vi "main_prepare_run.vi"(6 "Meth. Path":refnum<vi>, 7 "Runtime":refnum<vi>, 9 "Hydr. Path":refnum<vi>, 10 "Runtime String":refnum<vi>, 11 "Env. Dir":refnum<vi>) -> ()   [LabVIEW 2019]
uses:
  lib/libSimulationControl/libSimulationControl.lvlib
panel:
  # "*******************************************************************\nBiogas Plant Control\n\nAuthor: Paul Zügel\nGCSC-Frankfurt am Main 2020\n\n*******************************************************************"
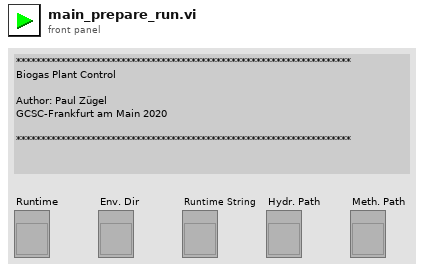
[diagram p1: front panel]
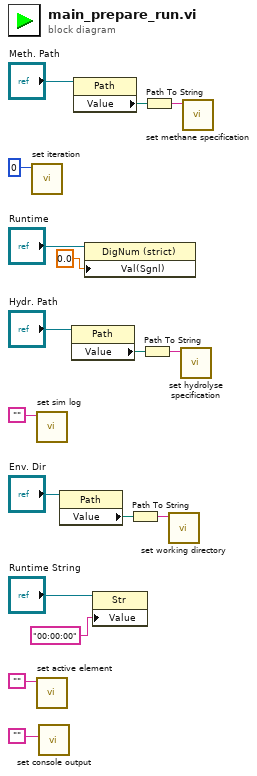
[diagram p0: block diagram]
diagram:
  n1 = call "set iteration.vi"("iter"=0 ("Value")) -> ()  [unwired: 10 in, 1 out]
  n2 = call "set sim log.vi"("log"="") -> ()  [unwired: 10 in, 1 out]
  n3 = call "set active element.vi"("elem"="") -> ()  [unwired: 10 in, 1 out]
  n4 = call "set console output.vi"("console_output"="") -> ()  [unwired: 11 in]
  n5 = property class="Path"(reference="Env. Dir") -> ("Value"=w16:path)  [unwired: 1 in, 2 out]
  n6 = property class="Path"(reference="Hydr. Path") -> ("Value"=w12:path)  [unwired: 1 in, 2 out]
  n7 = property class="Path"(reference="Meth. Path") -> ("Value"=w14:path)  [unwired: 1 in, 2 out]
  n8 = property on="Property Node" class="DigNum (strict)"(reference="Runtime", "Val(Sgnl)"=0.0 ("Value (Signaling)")) -> ()  [unwired: 1 in, 2 out]
  n9 = property on="Property Node" class="Str"(reference="Runtime String", "Value"="00:00:00") -> ()  [unwired: 1 in, 2 out]
  n10 = Path To String(path=w16) -> (string=w17:string)
  n11 = Path To String(path=w12) -> (string=w13:string)
  n12 = Path To String(path=w14) -> (string=w15:string)
  n13 = call "set working directory.vi"("dir"=w17) -> ()  [unwired: 10 in, 1 out]
  n14 = call "set hydrolyse specification.vi"("hydrolyse_spec_file"=w13) -> ()  [unwired: 10 in, 1 out]
  n15 = call "set methane specification.vi"("methane_spec_file"=w15) -> ()  [unwired: 10 in, 1 out]
